vi "load.vi"(8 "error in (no error)":errorcluster, 10 "child node in":refnum<k20>, 11 "Counter in":refnum<class "Counter.lvclass">) -> (0 "error out":errorcluster, 2 "child node out":refnum<k20>, 3 "Counter out":refnum<class "Counter.lvclass">)   [LabVIEW 2014, in "Counter.lvclass"]
uses:
  Counter.lvclass
  Counter.lvclass/Counter.ctl
  Globals.vi
  <vilib>/xml/Close Reference(Node).vi
  <resource>/objmgr/DOMUserDefRef.rc
  <vilib>/xml/NI_XML.lvlib
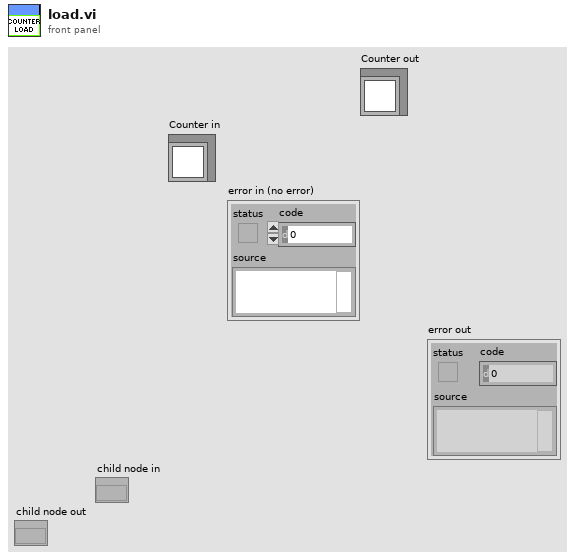
[diagram p1: front panel]
types:
  T1 = cluster{"Counter Channel":tag, "Time-Bin Clock Channel":tag, "Binwidth (ms)":dbl}
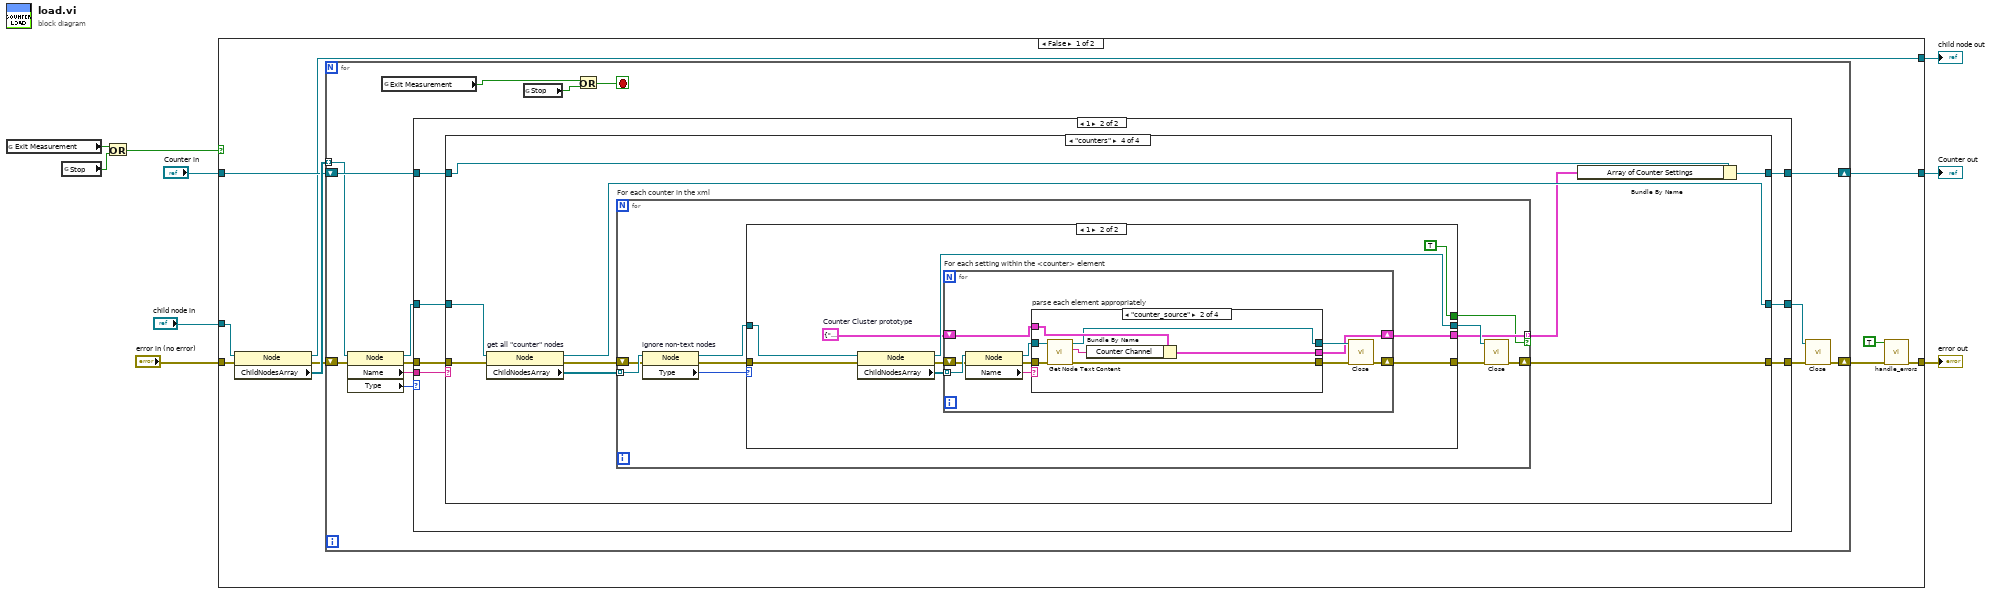
[diagram p0: block diagram]
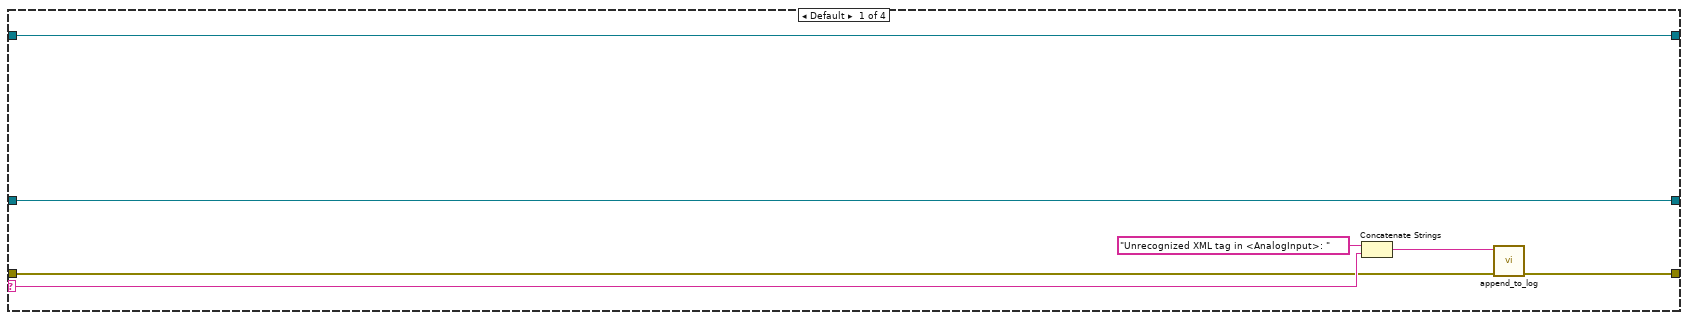
[diagram p3: hidden frame]
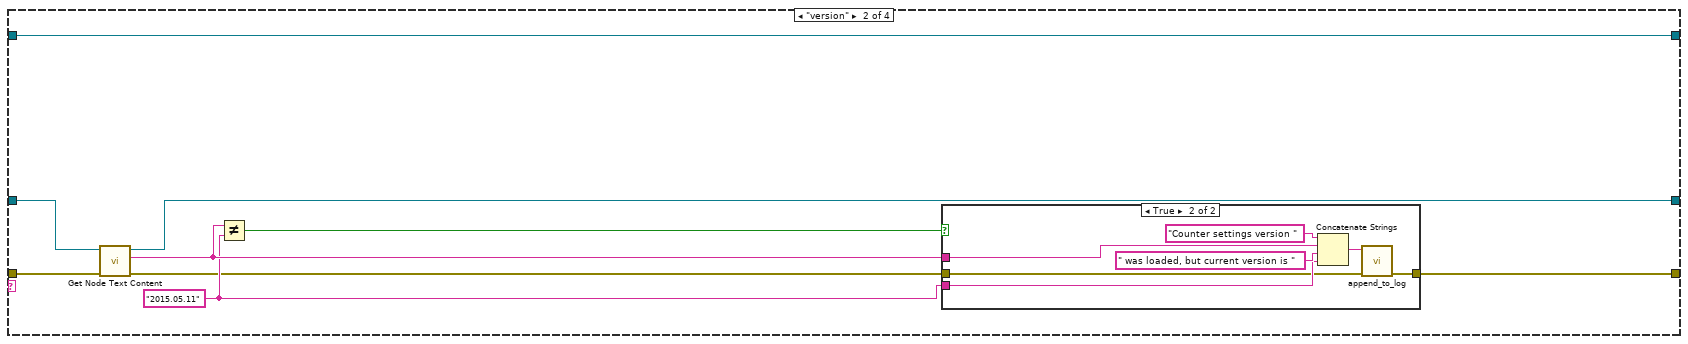
[diagram p4: hidden frame]
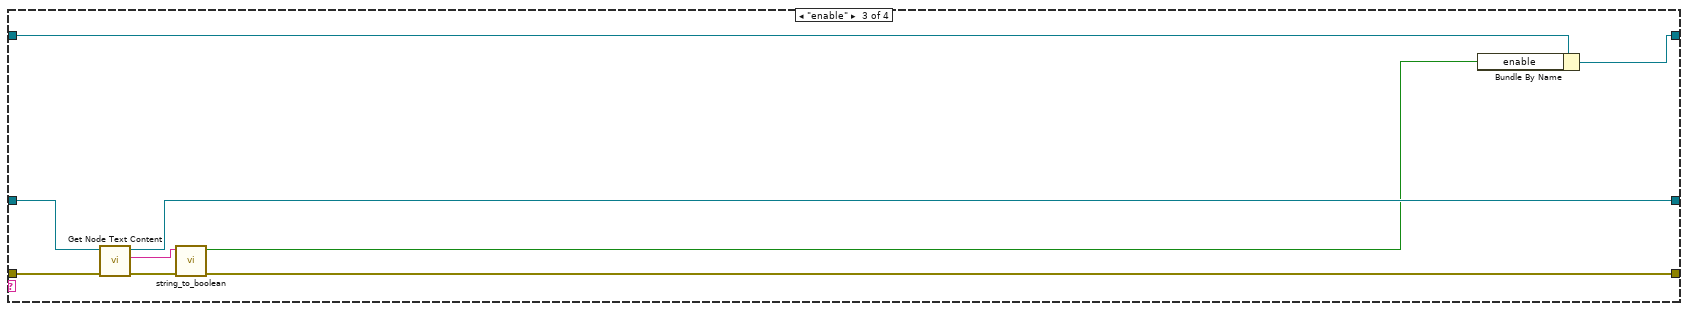
[diagram p6: hidden frame]
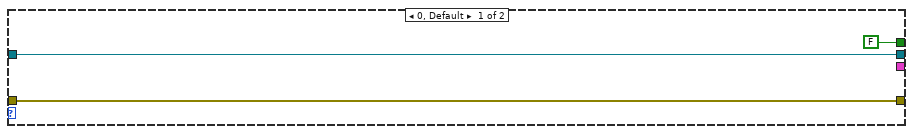
[diagram p7: hidden frame]
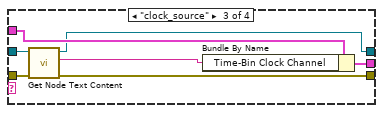
[diagram p9: hidden frame]
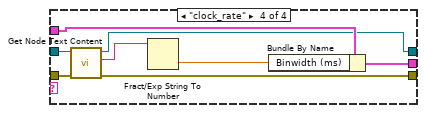
[diagram p10: hidden frame]
diagram:
  n1 = global read "Globals.vi" "Exit Measurement"() -> (w9:bool)
  n2 = global read "Globals.vi" "Stop"() -> (w8:bool)
  n3 = Or(x=w9, y=w8) -> (x .or. y?=w7:bool)
  n4 = case shown="False" w7 {
    tunnel: [w18 w145] -> w3
    tunnel: "error in (no error)" -> [w19 w145]
    tunnel: "Counter in" -> [w13 w144]
    tunnel: [w12 w144] -> w1
    tunnel: "child node in" -> [w11 w143]
    tunnel: [w10 w143] -> w5
    frame False {
      n5 = property class="Node"(reference=w11, error in=w19) -> (reference out=w10:refnum<k20>, error out=w16:errorcluster, "ChildNodesArray"=w17:refnum<k20>[])
      n6 = for {
        tunnel: w17 -> [w24] mode=indexing
        shift-right: [w30] -> w12
        shift-left: w13 -> [w31]
        shift-right: [w27] -> w15
        shift-left: w16 -> [w25]
        stop <- w20 stop-if-true
        n7 = property class="Node"(reference=w24, error in=w25) -> (reference out=w32:refnum<k20>, error out=w28:errorcluster, "Name"=w33:string, "Type"=w23:i32)
        n8 = global read "Globals.vi" "Exit Measurement"() -> (w22:bool)
        n9 = case shown="1" w23 {
          tunnel: w33 -> [_ w43]
          tunnel: w32 -> [w36 w42]
          tunnel: w31 -> [w34 w41]
          tunnel: [w34 w40] -> w30
          tunnel: [w36 w39] -> w29
          tunnel: w28 -> [w35 w38]
          tunnel: [w35 w37] -> w26
          frame Default {
          }
          frame 1 {
            n10 = case shown="\"counters\"" w43 {
              selector: w43 -> [w46 _ _ _]
              tunnel: w42 -> [w49 w54 w75 w81]
              tunnel: w41 -> [w50 w53 w73 w85]
              tunnel: [w50 w53 w72 w84] -> w40
              tunnel: [w49 w52 w76 w79] -> w39
              tunnel: w38 -> [w45 w55 w74 w80]
              tunnel: [w44 w51 w68 w78] -> w37
              frame Default {
                n11 = Concatenate Strings("Unrecognized XML tag in <AnalogInput>: " ("string"), w46) -> (w47:string)
                n12 = call "append_to_log.vi"("error in"=w45, "string"=w47) -> ("error out"=w44:errorcluster)  [unwired: 9 in]
              }
              frame "version" {
                w57 = "2015.05.11" ("y")
                n13 = call <vilib>:"Get Node Text Content.vi"("error in (no error)"=w55, "node in"=w54) -> ("error out"=w56:errorcluster, "node text"=w58:string, "node out"=w52:refnum<k20>)  [unwired: 7 in]
                n14 = Not Equal?(x=w58, y=w57) -> (x != y?=w59:bool)
                n15 = case shown="True" w59 {
                  tunnel: w58 -> [_ w66]
                  tunnel: w57 -> [_ w64]
                  tunnel: w56 -> [w60 w62]
                  tunnel: [w60 w61] -> w51
                  frame False {
                  }
                  frame True {
                    n16 = Concatenate Strings("Counter settings version " ("string"), w66, " was loaded, but current version is " ("string"), w64) -> (w63:string)
                    n17 = call "append_to_log.vi"("error in"=w62, "string"=w63) -> ("error out"=w61:errorcluster)  [unwired: 9 in]
                  }
                }
              }
              frame "enable" {
                n18 = call <vilib>:"Get Node Text Content.vi"("error in (no error)"=w74, "node in"=w75) -> ("error out"=w70:errorcluster, "node text"=w71:string, "node out"=w76:refnum<k20>)  [unwired: 7 in]
                n19 = call "string_to_boolean.vi"("error in"=w70, "string"=w71) -> ("error out"=w68:errorcluster, "boolean"=w69:bool)  [unwired: 8 in]
                n20 = Bundle By Name(cluster=w73, "enable"=w69) -> (w72:refnum<class "Counter.lvclass">)
              }
              frame "counters" {
                n21 = property on="get all \"counter\" nodes" class="Node"(reference=w81, error in=w80) -> (reference out=w79:refnum<k20>, error out=w82:errorcluster, "ChildNodesArray"=w83:refnum<k20>[])
                n22 = for "For each counter in the xml" {
                  tunnel: w83 -> [w91] mode=indexing
                  shift-right: [w95] -> w78
                  shift-left: w82 -> [w88]
                  tunnel: [w92] -> w77 mode=indexing if=w86
                  n23 = property on="ignore non-text nodes" class="Node"(reference=w91, error in=w88) -> (reference out=w90:refnum<k20>, error out=w87:errorcluster, "Type"=w89:i32)
                  n24 = case shown="1" w89 {
                    tunnel: w90 -> [w97 w107]
                    tunnel: w87 -> [w98 w105]
                    tunnel: [w97 w103] -> w94
                    tunnel: [w98 w102] -> w93
                    tunnel: [_ w100] -> w92
                    tunnel: [FALSE TRUE] -> w86
                    frame 0, Default {
                    }
                    frame 1 {
                      w101 = T1 {"Counter Channel"="", "Time-Bin Clock Channel"="", "Binwidth (ms)"=0.0}  # Counter Cluster prototype
                      n25 = property class="Node"(reference=w107, error in=w105) -> (reference out=w103:refnum<k20>, error out=w104:errorcluster, "ChildNodesArray"=w106:refnum<k20>[])
                      n26 = for "For each setting within the <counter> element" {
                        tunnel: w106 -> [w117] mode=indexing
                        shift-right: [w112] -> w102
                        shift-left: w104 -> [w115]
                        shift-right: [w108] -> w100
                        shift-left: w101 -> [w110]
                        n27 = property class="Node"(reference=w117, error in=w115) -> (reference out=w111:refnum<k20>, error out=w114:errorcluster, "Name"=w116:string)
                        n28 = case "parse each element appropriately" shown="\"counter_source\"" w116 {
                          tunnel: w114 -> [w120 w126 w133 w141]
                          tunnel: [w120 w123 w130 w139] -> w113
                          tunnel: w111 -> [w119 w127 w134 w142]
                          tunnel: w110 -> [w118 w125 w132 w140]
                          tunnel: [w119 w122 w129 w138] -> w109
                          tunnel: [w118 w121 w128 w135] -> w108
                          frame "None", Default {
                          }
                          frame "counter_source" {
                            n29 = call <vilib>:"Get Node Text Content.vi"("error in (no error)"=w126, "node in"=w127) -> ("error out"=w123:errorcluster, "node text"=w124:string, "node out"=w122:refnum<k20>)  [unwired: 7 in]
                            n30 = Bundle By Name(cluster=w125, "Counter Channel"=w124) -> (w121:T1)
                          }
                          frame "clock_source" {
                            n31 = call <vilib>:"Get Node Text Content.vi"("error in (no error)"=w133, "node in"=w134) -> ("error out"=w130:errorcluster, "node text"=w131:string, "node out"=w129:refnum<k20>)  [unwired: 7 in]
                            n32 = Bundle By Name(cluster=w132, "Time-Bin Clock Channel"=w131) -> (w128:T1)
                          }
                          frame "clock_rate" {
                            n33 = call <vilib>:"Get Node Text Content.vi"("error in (no error)"=w141, "node in"=w142) -> ("error out"=w139:errorcluster, "node text"=w137:string, "node out"=w138:refnum<k20>)  [unwired: 7 in]
                            n34 = Fract/Exp String To Number(string=w137) -> (number=w136:dbl)  [unwired: 3 in, 1 out]
                            n35 = Bundle By Name(cluster=w140, "Binwidth (ms)"=w136) -> (w135:T1)
                          }
                        }
                        n36 = call-poly <vilib>:"Close.vi"("error in (no error)"=w113, "node"=w109) -> ("error out"=w112:errorcluster)  [unwired: 7 in]
                      }
                    }
                  }
                  n37 = call-poly <vilib>:"Close.vi"("error in (no error)"=w93, "node"=w94) -> ("error out"=w95:errorcluster)  [unwired: 7 in]
                }
                n38 = Bundle By Name(cluster=w85, "Array of Counter Settings"=w77) -> (w84:refnum<class "Counter.lvclass">)
              }
            }
          }
        }
        n39 = global read "Globals.vi" "Stop"() -> (w21:bool)
        n40 = Or(x=w22, y=w21) -> (x .or. y?=w20:bool)
        n41 = call-poly <vilib>:"Close.vi"("error in (no error)"=w26, "node"=w29) -> ("error out"=w27:errorcluster)  [unwired: 7 in]
      }
      n42 = call "handle_errors.vi"("Exit Operation"=TRUE, "error in (no error)"=w15) -> ("error out"=w18:errorcluster)  [unwired: 13 in]
    }
    frame True {
    }
  }
  "error out" <- w3
  "Counter out" <- w1
  "child node out" <- w5
